vi "turn_.vi"(9 "delay":u32, 10 "Carzeta":dbl) -> ()   [LabVIEW 2017]
uses:
  GlobalVar.vi
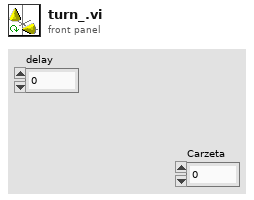
[diagram p1: front panel]
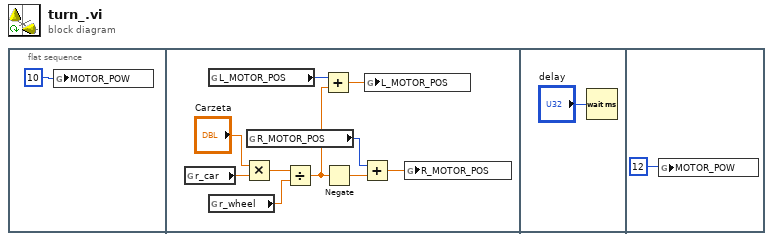
[diagram p0: block diagram]
diagram:
  n1 = flat-sequence {
    frame #0 {
      n2 = global write "GlobalVar.vi" "MOTOR_POW"(i8 10 ("MOTOR_POW")) -> ()
    }
    frame #1 {
      n3 = global read "GlobalVar.vi" "r_car"() -> (w4:dbl)
      n4 = global read "GlobalVar.vi" "L_MOTOR_POS"() -> (w9:i32)
      n5 = global read "GlobalVar.vi" "r_wheel"() -> (w5:dbl)
      n6 = Multiply(x="Carzeta", y=w4) -> (x*y=w10:dbl)
      n7 = global read "GlobalVar.vi" "R_MOTOR_POS"() -> (w8:i32)
      n8 = Divide(x=w10, y=w5) -> (x/y=w2:dbl)
      n9 = Add(x=w9, y=w2) -> (x+y=w7:dbl)
      n10 = Negate(x=w2) -> (-x=w3:dbl)
      n11 = Add(x=w8, y=w3) -> (x+y=w6:dbl)
      n12 = global write "GlobalVar.vi" "L_MOTOR_POS"(w7) -> ()
      n13 = global write "GlobalVar.vi" "R_MOTOR_POS"(w6) -> ()
    }
    frame #2 {
      n14 = Wait (ms)(milliseconds to wait="delay") -> ()  [unwired: 1 out]
    }
    frame #3 {
      n15 = global write "GlobalVar.vi" "MOTOR_POW"(i8 12 ("MOTOR_POW")) -> ()
    }
  }
